vi "4.3.vi"() -> ()   [LabVIEW 2017]
panel:
  out "平均值":dbl
  in  "输入值":dbl
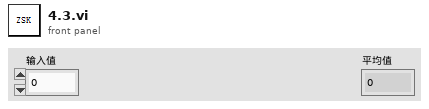
[diagram p1: front panel]
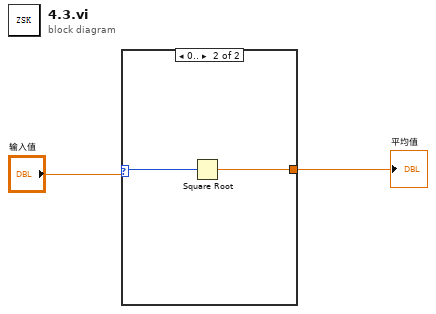
[diagram p0: block diagram]
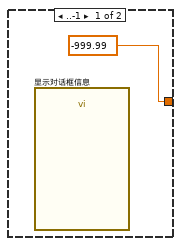
[diagram p2: hidden frame]
diagram:
  n1 = case shown="0.." "输入值" {
    selector: "输入值" -> [_ w5]
    tunnel: [-999.99 w4] -> w1
    frame ..-1 {
      n2 = call "显示对话框信息"() -> ()  [unwired: 10 in, 2 out]
    }
    frame 0.. {
      n3 = Square Root(x=w5) -> (sqrt(x)=w4:dbl)
    }
  }
  "平均值" <- w1
